vi "Buffer_Initialize.vi"(8 "error in (no error)":errorcluster, 11 "DataCluster in":T1={"Core"={"Current VI Reference"=refnum, "Close Panel on Exit?"=FALSE, "Exit"=FALSE, "Initialized?"=FALSE}, "Connections"={"cDAQ DO"={"Task"="", "Connected"=FALSE, "Active"=FALSE, "ID"=""}, "cDAQ AO"={"Task"="", "Connected"=FALSE, "Active"=FALSE, "ID"=""}, "cDAQ AI"={"Task"="", "Connected"=FALSE, "Active"=FALSE, "ID"=""}, "Camera"={"Session"="", "Connected"=FALSE, "Active"=FALSE, "Placeholder"=refnum}, "Humidity"={"Port"="", "Connected"=FALSE, "Active"=FALSE}}, "Data Acquisition"={"Setup"={"Label"="", "Operator"="", "Notes"="", "CircTemp"=1.0, "FlowRate"=1.0}, "Camera"={"Image"=refnum, "Save Image"=refnum, "Image Frequency"=20, "Rectangle"={"Left"=0, "Top"=0, "Right"=0, "Bottom"=0, "Rotation"=0.0}, "Calibration"={"Top Left"={"X"=0.0, "Y"=0.0}, "Top Right"={"X"=0.0, "Y"=0.0}, "Bottom Left"={"X"=0.0, "Y"=0.0}, "Bottom Right"={"X"=0.0, "Y"=0.0}, "Fixpoint"={"X"=0.0, "Y"=0.0}, "Scan Area"=0.0, "Fixpoint Area"=0.0, "Well Pixels"=[], "Valid"=FALSE}, "FocusPos"=0, "Display Mapping"=10}, "Thermistor"={"Sample Size"=1, "Calibration"={"B0.100"=[], "R25"=[], "c"=[], "State"=[], "V_S"=5.0, "R_S"=100.0}, "Timing Mode"=14713}, "Partition"={"Data"=[], "Cell Label"="", "Cell Color"=0, "Height"=10, "Width"=16, "Grid"=[]}, "Queue"={"Queue"=refnum, "Size"=1}, "Sample Rate"=20, "Active"=FALSE, "Ready"=FALSE, "Graph Mode"=0, "Gradient Buffer"=2, "DC Auto"=FALSE}, "Control"={"Sample Rate"=1, "LogStart ms"=0, "AC PSU"={"Voltage"=0.0, "Frequency"=0.0, "State"={"15+16 - Waveform"=0, "17 - Freq Control EN"=FALSE, "18 - Voltage Output"=FALSE, "19 - Output Mode"=0, "20 - Mode Control EN"=FALSE, "21 - AC Control EN"=FALSE, "24 - DC Control EN"=FALSE, "25 - DC Polarity Bias"=FALSE}}, "DC PSU"={"Voltage"=0.0, "Active"=FALSE, "Pulse Size"=0.0, "Pulse Duration"=0.0, "Voltage Set"=0.0}, "Computer Vision"={"Target Pos"=0.0, "Current Pos"=0.0, "Processing"=refnum, "Range"={"Lower value"=128.0, "Upper value"=255.0}, "MinArea"=2, "16-bit Conversion Method"=10, "Display Image"=10, "Binary"=refnum, "Gain"=0.0, "Exposure time"=0.0}, "PID"={"AutoPID"=FALSE, "Gains"={"proportional gain (Kc)"=1.0, "integral time (Ti, min)"=0.01, "derivative time (Td, min)"=0.0}, "autotuning parameters"={"controller type"=1, "relay cycles"=3, "relay amplitude"=1.0, "control specification"=2, "PV noise level"=0.1}, "Show Controls"=FALSE}}, "Manual Temp Control"={"TargetTemp"=1.0, "Mode"=0, "Active"=FALSE}} {"Manual Temp Control"."Mode" items=["Cool", "Heat"]; "Manual Temp Control"."TargetTemp" min=-40.0 max=40.0 step=0.5 format="%#_g °C"; "Control"."PID"."autotuning parameters"."PV noise level" format="%.2f"; "Control"."PID"."autotuning parameters"."control specification" items=["normal", "fast", "slow"]; "Control"."PID"."autotuning parameters"."relay amplitude" format="%.2f"; "Control"."PID"."autotuning parameters"."controller type" items=["PID", "PI", "P"]; "Control"."PID"."Gains"."derivative time (Td, min)" format="%.3f"; "Control"."PID"."Gains"."integral time (Ti, min)" format="%.3f"; "Control"."PID"."Gains"."proportional gain (Kc)" format="%.3f"; "Control"."Computer Vision"."Display Image" items=["Default", "Computer Vision"]; "Control"."Computer Vision"."16-bit Conversion Method" items=["Default"=10, "Most Significant Bits"=11, "Full Dynamic"=12, "Downshift"=13, "Given Range"=14, "90% Dynamic"=15, "Given Percent Range"=16]; "Control"."Computer Vision"."Range"."Upper value" format="%.2f"; "Control"."Computer Vision"."Range"."Lower value" format="%.2f"; "Control"."AC PSU"."State"."19 - Output Mode" items=["Constant Voltage", "Constant Current"]; "Control"."AC PSU"."State"."15+16 - Waveform" items=["Sine", "Square", "Triangle"]; "Control"."Sample Rate" min=1 max=20 step=1 format="%.0f Samples/sec"; "Data Acquisition"."Gradient Buffer" min=2 max=30 step=1; "Data Acquisition"."Graph Mode" items=["Thermistor Temperature", "Camera Temperature"]; "Data Acquisition"."Thermistor"."Timing Mode" items=["Automatic"=16097, "High Resolution"=10195, "High Speed"=14712, "Best 50 Hz Rejection"=14713, "Best 60 Hz Rejection"=14714, "Custom"=10137]; "Data Acquisition"."Thermistor"."Calibration"."R_S" min=0.1 max=1000.0 format="%#_g kOhm"; "Data Acquisition"."Thermistor"."Calibration"."V_S" min=5.0 max=48.0 format="%#_g V"; "Data Acquisition"."Thermistor"."Calibration"."R25" min=0.1 max=1000.0 format="%#_g kOhm"; "Data Acquisition"."Thermistor"."Calibration"."B0.100" min=100.0 max=10000.0 format="%#_g K"; "Data Acquisition"."Thermistor"."Sample Size" min=1 max=200; "Data Acquisition"."Sample Rate" min=20 max=240 format="%.0f samples/min"; "Data Acquisition"."Queue"."Size" min=1 max=200; "Data Acquisition"."Camera"."Display Mapping" items=["Default"=10, "Most Significant Bits"=11, "Full Dynamic"=12, "Downshift"=13, "Given Range"=14, "90% Dynamic"=15, "Given Percent Range"=16]; "Data Acquisition"."Camera"."Calibration"."Fixpoint"."Y" format="%.2f"; "Data Acquisition"."Camera"."Calibration"."Fixpoint"."X" format="%.2f"; "Data Acquisition"."Camera"."Calibration"."Top Left"."Y" format="%.2f"; "Data Acquisition"."Camera"."Calibration"."Top Left"."X" format="%.2f"; "Data Acquisition"."Camera"."Calibration"."Top Right"."Y" format="%.2f"; "Data Acquisition"."Camera"."Calibration"."Top Right"."X" format="%.2f"; "Data Acquisition"."Camera"."Calibration"."Bottom Left"."Y" format="%.2f"; "Data Acquisition"."Camera"."Calibration"."Bottom Left"."X" format="%.2f"; "Data Acquisition"."Camera"."Calibration"."Bottom Right"."Y" format="%.2f"; "Data Acquisition"."Camera"."Calibration"."Bottom Right"."X" format="%.2f"; "Data Acquisition"."Camera"."Rectangle"."Rotation" min=-90.0 max=90.0 step=1.0 format="%.2f"; "Data Acquisition"."Camera"."Rectangle"."Left" scale=0.0..1024.0; "Data Acquisition"."Camera"."Rectangle"."Right" scale=0.0..1024.0; "Data Acquisition"."Camera"."Image Frequency" min=1 max=60 step=1; "Data Acquisition"."Setup"."FlowRate" min=0.0 max=500.0 format="%#_g L/min"; "Data Acquisition"."Setup"."CircTemp" min=-40.0 max=40.0 step=0.5 format="%#_g °C"}) -> (0 "error out":errorcluster, 3 "DataCluster Out":T1={"Core"={"Current VI Reference"=refnum, "Close Panel on Exit?"=FALSE, "Exit"=FALSE, "Initialized?"=FALSE}, "Connections"={"cDAQ DO"={"Task"="", "Connected"=FALSE, "Active"=FALSE, "ID"=""}, "cDAQ AO"={"Task"="", "Connected"=FALSE, "Active"=FALSE, "ID"=""}, "cDAQ AI"={"Task"="", "Connected"=FALSE, "Active"=FALSE, "ID"=""}, "Camera"={"Session"="", "Connected"=FALSE, "Active"=FALSE, "Placeholder"=refnum}, "Humidity"={"Port"="", "Connected"=FALSE, "Active"=FALSE}}, "Data Acquisition"={"Setup"={"Label"="", "Operator"="", "Notes"="", "CircTemp"=1.0, "FlowRate"=1.0}, "Camera"={"Image"=refnum, "Save Image"=refnum, "Image Frequency"=20, "Rectangle"={"Left"=0, "Top"=0, "Right"=0, "Bottom"=0, "Rotation"=0.0}, "Calibration"={"Top Left"={"X"=0.0, "Y"=0.0}, "Top Right"={"X"=0.0, "Y"=0.0}, "Bottom Left"={"X"=0.0, "Y"=0.0}, "Bottom Right"={"X"=0.0, "Y"=0.0}, "Fixpoint"={"X"=0.0, "Y"=0.0}, "Scan Area"=0.0, "Fixpoint Area"=0.0, "Well Pixels"=[], "Valid"=FALSE}, "FocusPos"=0, "Display Mapping"=10}, "Thermistor"={"Sample Size"=1, "Calibration"={"B0.100"=[], "R25"=[], "c"=[], "State"=[], "V_S"=5.0, "R_S"=100.0}, "Timing Mode"=14713}, "Partition"={"Data"=[], "Cell Label"="", "Cell Color"=0, "Height"=10, "Width"=16, "Grid"=[]}, "Queue"={"Queue"=refnum, "Size"=1}, "Sample Rate"=20, "Active"=FALSE, "Ready"=FALSE, "Graph Mode"=0, "Gradient Buffer"=2, "DC Auto"=FALSE}, "Control"={"Sample Rate"=1, "LogStart ms"=0, "AC PSU"={"Voltage"=0.0, "Frequency"=0.0, "State"={"15+16 - Waveform"=0, "17 - Freq Control EN"=FALSE, "18 - Voltage Output"=FALSE, "19 - Output Mode"=0, "20 - Mode Control EN"=FALSE, "21 - AC Control EN"=FALSE, "24 - DC Control EN"=FALSE, "25 - DC Polarity Bias"=FALSE}}, "DC PSU"={"Voltage"=0.0, "Active"=FALSE, "Pulse Size"=0.0, "Pulse Duration"=0.0, "Voltage Set"=0.0}, "Computer Vision"={"Target Pos"=0.0, "Current Pos"=0.0, "Processing"=refnum, "Range"={"Lower value"=128.0, "Upper value"=255.0}, "MinArea"=2, "16-bit Conversion Method"=10, "Display Image"=10, "Binary"=refnum, "Gain"=0.0, "Exposure time"=0.0}, "PID"={"AutoPID"=FALSE, "Gains"={"proportional gain (Kc)"=1.0, "integral time (Ti, min)"=0.01, "derivative time (Td, min)"=0.0}, "autotuning parameters"={"controller type"=1, "relay cycles"=3, "relay amplitude"=1.0, "control specification"=2, "PV noise level"=0.1}, "Show Controls"=FALSE}}, "Manual Temp Control"={"TargetTemp"=1.0, "Mode"=0, "Active"=FALSE}} {"Manual Temp Control"."Mode" items=["Cool", "Heat"]; "Manual Temp Control"."TargetTemp" min=-40.0 max=40.0 step=0.5 format="%#_g °C"; "Control"."PID"."autotuning parameters"."PV noise level" format="%.2f"; "Control"."PID"."autotuning parameters"."control specification" items=["normal", "fast", "slow"]; "Control"."PID"."autotuning parameters"."relay amplitude" format="%.2f"; "Control"."PID"."autotuning parameters"."controller type" items=["PID", "PI", "P"]; "Control"."PID"."Gains"."derivative time (Td, min)" format="%.3f"; "Control"."PID"."Gains"."integral time (Ti, min)" format="%.3f"; "Control"."PID"."Gains"."proportional gain (Kc)" format="%.3f"; "Control"."Computer Vision"."Display Image" items=["Default", "Computer Vision"]; "Control"."Computer Vision"."16-bit Conversion Method" items=["Default"=10, "Most Significant Bits"=11, "Full Dynamic"=12, "Downshift"=13, "Given Range"=14, "90% Dynamic"=15, "Given Percent Range"=16]; "Control"."Computer Vision"."Range"."Upper value" format="%.2f"; "Control"."Computer Vision"."Range"."Lower value" format="%.2f"; "Control"."AC PSU"."State"."19 - Output Mode" items=["Constant Voltage", "Constant Current"]; "Control"."AC PSU"."State"."15+16 - Waveform" items=["Sine", "Square", "Triangle"]; "Control"."Sample Rate" min=1 max=20 step=1 format="%.0f Samples/sec"; "Data Acquisition"."Gradient Buffer" min=2 max=30 step=1; "Data Acquisition"."Graph Mode" items=["Thermistor Temperature", "Camera Temperature"]; "Data Acquisition"."Thermistor"."Timing Mode" items=["Automatic"=16097, "High Resolution"=10195, "High Speed"=14712, "Best 50 Hz Rejection"=14713, "Best 60 Hz Rejection"=14714, "Custom"=10137]; "Data Acquisition"."Thermistor"."Calibration"."R_S" min=0.1 max=1000.0 format="%#_g kOhm"; "Data Acquisition"."Thermistor"."Calibration"."V_S" min=5.0 max=48.0 format="%#_g V"; "Data Acquisition"."Thermistor"."Calibration"."R25" min=0.1 max=1000.0 format="%#_g kOhm"; "Data Acquisition"."Thermistor"."Calibration"."B0.100" min=100.0 max=10000.0 format="%#_g K"; "Data Acquisition"."Thermistor"."Sample Size" min=1 max=200; "Data Acquisition"."Sample Rate" min=20 max=240 format="%.0f samples/min"; "Data Acquisition"."Queue"."Size" min=1 max=200; "Data Acquisition"."Camera"."Display Mapping" items=["Default"=10, "Most Significant Bits"=11, "Full Dynamic"=12, "Downshift"=13, "Given Range"=14, "90% Dynamic"=15, "Given Percent Range"=16]; "Data Acquisition"."Camera"."Calibration"."Fixpoint"."Y" format="%.2f"; "Data Acquisition"."Camera"."Calibration"."Fixpoint"."X" format="%.2f"; "Data Acquisition"."Camera"."Calibration"."Top Left"."Y" format="%.2f"; "Data Acquisition"."Camera"."Calibration"."Top Left"."X" format="%.2f"; "Data Acquisition"."Camera"."Calibration"."Top Right"."Y" format="%.2f"; "Data Acquisition"."Camera"."Calibration"."Top Right"."X" format="%.2f"; "Data Acquisition"."Camera"."Calibration"."Bottom Left"."Y" format="%.2f"; "Data Acquisition"."Camera"."Calibration"."Bottom Left"."X" format="%.2f"; "Data Acquisition"."Camera"."Calibration"."Bottom Right"."Y" format="%.2f"; "Data Acquisition"."Camera"."Calibration"."Bottom Right"."X" format="%.2f"; "Data Acquisition"."Camera"."Rectangle"."Rotation" min=-90.0 max=90.0 step=1.0 format="%.2f"; "Data Acquisition"."Camera"."Rectangle"."Left" scale=0.0..1024.0; "Data Acquisition"."Camera"."Rectangle"."Right" scale=0.0..1024.0; "Data Acquisition"."Camera"."Image Frequency" min=1 max=60 step=1; "Data Acquisition"."Setup"."FlowRate" min=0.0 max=500.0 format="%#_g L/min"; "Data Acquisition"."Setup"."CircTemp" min=-40.0 max=40.0 step=0.5 format="%#_g °C"})   [LabVIEW 2024]
uses:
  DataCluster.ctl
  <vilib>/userDefined/High Color/IMAQdx.ctl
  <vilib>/vision/Image Controls.llb/IMAQ Image.ctl
  DataQueue.ctl
  SensorCluster.ctl
  DataCluster_AC_PSU.ctl
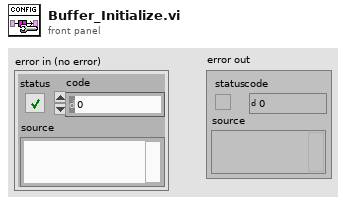
[diagram p1: front panel]
types:
  T1 = typedef "DataCluster.ctl" = cluster{"Core":cluster{"Current VI Reference":refnum<vi>, "Close Panel on Exit?":bool, "Exit":bool, "Initialized?":bool}, "Connections":cluster{"cDAQ DO":cluster{"Task":refnum<k21>, "Connected":bool, "Active":bool, "ID":string}, "cDAQ AO":cluster{"Task":refnum<k21>, "Connected":bool, "Active":bool, "ID":string}, "cDAQ AI":cluster{"Task":refnum<k21>, "Connected":bool, "Active":bool, "ID":string}, "Camera":cluster{"Session":T2, "Connected":bool, "Active":bool, "Placeholder":T3}, "Humidity":cluster{"Port":refnum<visa-resource-name>, "Connected":bool, "Active":bool}}, "Data Acquisition":cluster{"Setup":cluster{"Label":string, "Operator":string, "Notes":string, "CircTemp":dbl, "FlowRate":dbl}, "Camera":cluster{"Image":T3, "Save Image":T3, "Image Frequency":i32, "Rectangle":T4, "Calibration":cluster{"Top Left":T5, "Top Right":T5, "Bottom Left":T5, "Bottom Right":T5, "Fixpoint":T5, "Scan Area":dbl, "Fixpoint Area":dbl, "Well Pixels":cluster{"X":i32, "Y":i32}[][], "Valid":bool}, "FocusPos":u32, "Display Mapping":u32}, "Thermistor":cluster{"Sample Size":i32, "Calibration":cluster{"B0.100":dbl[], "R25":dbl[], "c":dbl[][], "State":bool[], "V_S":dbl, "R_S":dbl}, "Timing Mode":i32}, "Partition":cluster{"Data":string[][], "Cell Label":string, "Cell Color":u32, "Height":i32, "Width":i32, "Grid":string[][]}, "Queue":cluster{"Queue":refnum<queue>, "Size":i32}, "Sample Rate":i32, "Active":bool, "Ready":bool, "Graph Mode":u16, "Gradient Buffer":i32, "DC Auto":bool}, "Control":cluster{"Sample Rate":i32, "LogStart ms":u32, "AC PSU":cluster{"Voltage":dbl[unit], "Frequency":dbl[unit], "State":T6}, "DC PSU":cluster{"Voltage":dbl[unit], "Active":bool, "Pulse Size":dbl[unit], "Pulse Duration":dbl[unit], "Voltage Set":dbl[unit]}, "Computer Vision":cluster{"Target Pos":dbl, "Current Pos":dbl, "Processing":T3, "Range":cluster{"Lower value":sgl, "Upper value":sgl}, "MinArea":i32, "16-bit Conversion Method":u32, "Display Image":u32, "Binary":T3, "Gain":dbl, "Exposure time":dbl}, "PID":cluster{"AutoPID":bool, "Gains":cluster{"proportional gain (Kc)":dbl, "integral time (Ti, min)":dbl, "derivative time (Td, min)":dbl}, "autotuning parameters":cluster{"controller type":u16, "relay cycles":i32, "relay amplitude":dbl, "control specification":u16, "PV noise level":dbl}, "Show Controls":bool}}, "Manual Temp Control":cluster{"TargetTemp":dbl, "Mode":u16, "Active":bool}}
  T2 = typedef "IMAQdx.ctl" = refnum<k21>
  T3 = typedef "IMAQ Image.ctl" = refnum<image>
  T4 = typedef "IMAQ Rectangle" = cluster{"Left":i32, "Top":i32, "Right":i32, "Bottom":i32, "Rotation":dbl}
  T5 = typedef "IMAQ Point" = cluster{"X":sgl, "Y":sgl}
  T6 = typedef "DataCluster_AC_PSU.ctl" = cluster{"15+16 - Waveform":u16, "17 - Freq Control EN":bool, "18 - Voltage Output":bool, "19 - Output Mode":u16, "20 - Mode Control EN":bool, "21 - AC Control EN":bool, "24 - DC Control EN":bool, "25 - DC Polarity Bias":bool}
  T7 = typedef "DataQueue.ctl" = cluster{"Image Pixels (U16)":u16[][], "Current Time":string, "Sensor Cluster":T8}
  T8 = typedef "SensorCluster.ctl" = cluster{"Temp":dbl[unit], "AC V":dbl[unit], "AC Freq":dbl[unit], "DC V":dbl[unit], "Temp Readings":dbl[], "Voltage Readings":dbl[], "CMH":cluster{"Humidity":dbl, "Dewpoint":dbl, "Air Temp":dbl}, "Current Pos":dbl}
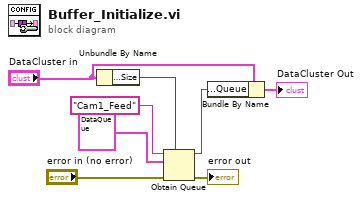
[diagram p0: block diagram]
diagram:
  n1 = Unbundle By Name("DataCluster in") -> ("Data Acquisition.Queue.Size"=w7:i32)
  n2 = Obtain Queue(max queue size (-1, unlimited)=w7, name (unnamed)="Cam1_Feed", element data type=T7 {"Image Pixels (U16)"=[], "Current Time"="", "Sensor Cluster"={"Temp"=0.0, "AC V"=0.0, "AC Freq"=0.0, "DC V"=0.0, "Temp Readings"=[], "Voltage Readings"=[], "CMH"={"Humidity"=0.0, "Dewpoint"=0.0, "Air Temp"=0.0}, "Current Pos"=0.0}} ("DataQueue"), error in (no error)="error in (no error)") -> (queue out=w1:refnum<queue>, error out=→"error out":errorcluster)  [unwired: 1 in, 1 out]
  n3 = Bundle By Name(cluster="DataCluster in", "Data Acquisition.Queue.Queue"=w1) -> (→"DataCluster Out":T1)
